vi "Data File Viewer.vi"(4 "error in (no error)":errorcluster, 6 "DataPlugin name":string, 7 "file path":path) -> (0 "error out":errorcluster, 2 "DataPlugin name out":string, 3 "file path out":path)   [LabVIEW 2020]
doc: "Opens the data file specified in the <B>file path</B> input and presents the data in the Data File Viewer dialog box."
uses:
  <vilib>/Utility/tdmsutil.llb/fileViewerConfigData.ctl
  <vilib>/Platform/storage/lvStorage.llb/_openFunction.ctl
  <vilib>/Platform/storage/Storage.llb/GetObjectFromID_Object.vi
panel:
  in  "Help":bool
  in  "Status":string
  in  "Quit":bool
  in  "Settings...":bool
  in  "Properties / Values / Graph":T1(tab)
  in  "Properties":i32(listbox)
  in  "Raw data values":i32(listbox)
  out "Waveform Graph":waveform(dbl)[](graph)
  in  "File contents":string(tree)
  # "Displaying values 1..1000"
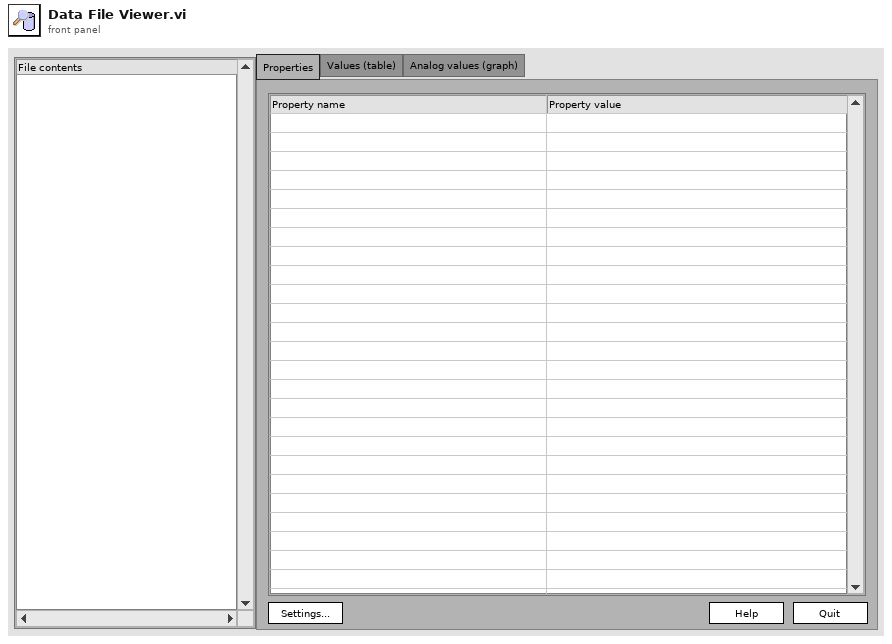
[diagram p1: front panel]
types:
  T1 = enum32{"Properties", "Values (table)", "Analog values (graph)"}
  T2 = typedef "_openFunction.ctl" = enum16{"open", "open or create", "create or replace", "create", "open (read only)"}
  T3 = typedef "fileViewerConfigData.ctl" = cluster{"Show all (table)":bool, "Show all (graph)":bool, "limit (table)":u64, "limit (graph)":u64, "no show":bool, "start (table)":u64, "start (graph)":u64}
  T4 = cluster{"Tree":refnum<vi>, "Tab Control":refnum<vi>, "property list":refnum<vi>, "raw data list":refnum<vi>, "Waveform Graph":refnum<vi>, "Ok":refnum<vi>, "Ok 2":refnum<vi>, "Ok 3":refnum<vi>, "Ok 4":refnum<vi>}
  T5 = typedef "usiPluginInformation.ctl" = cluster{"name":string, "version":string, "type":string, "read-only?":bool, "extensions":string[]}
  T6 = typedef "LVRectTypeDef.ctl" = cluster{"Left":i16, "Top":i16, "Right":i16, "Bottom":i16}
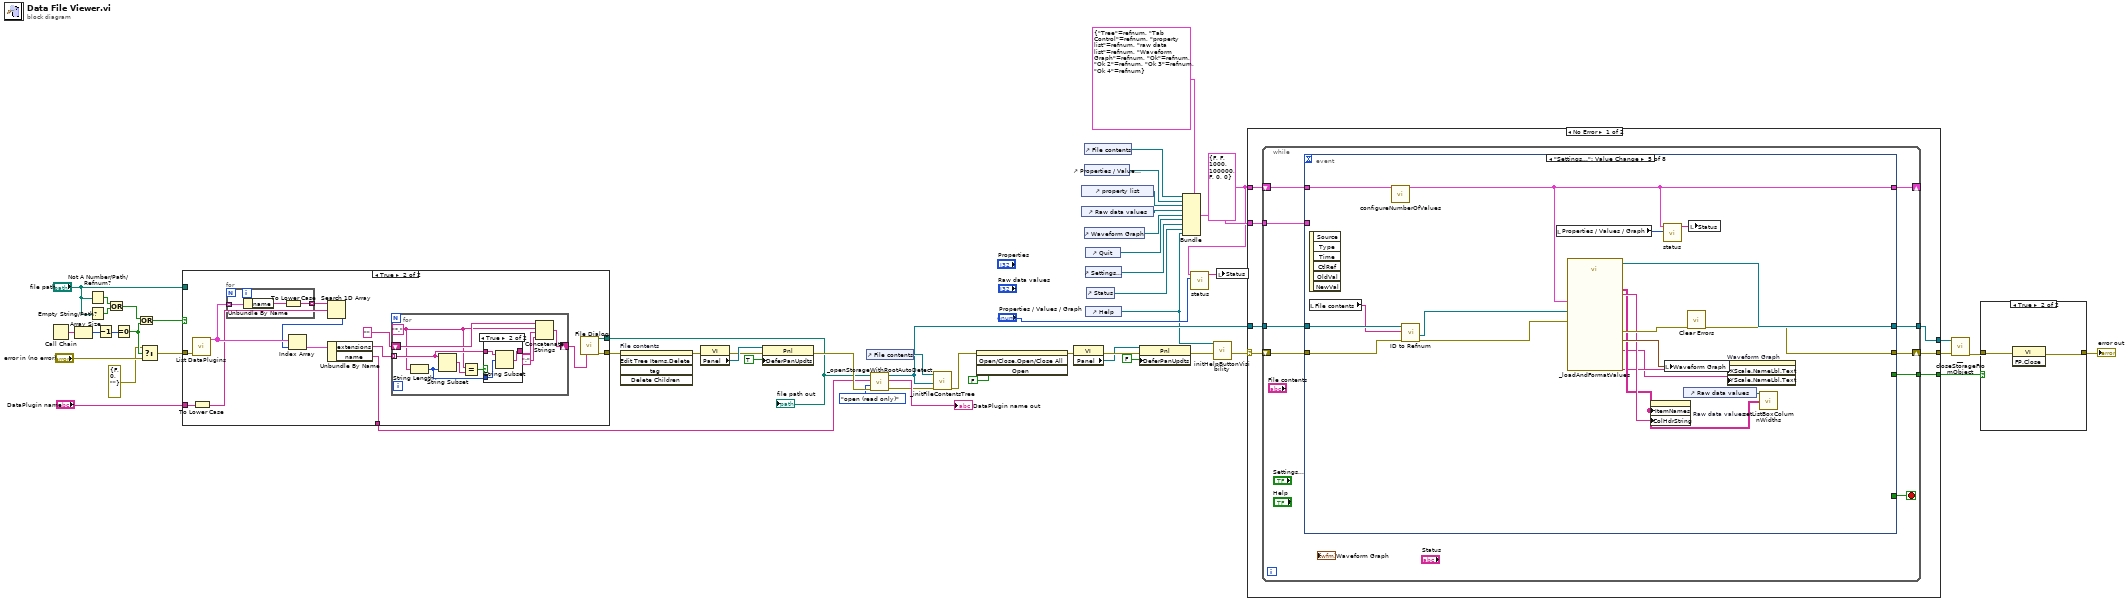
[diagram p0: block diagram]
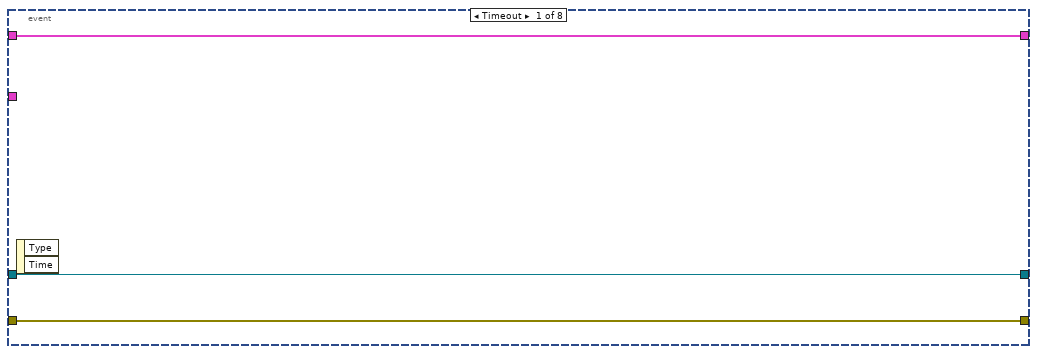
[diagram p5: hidden frame]
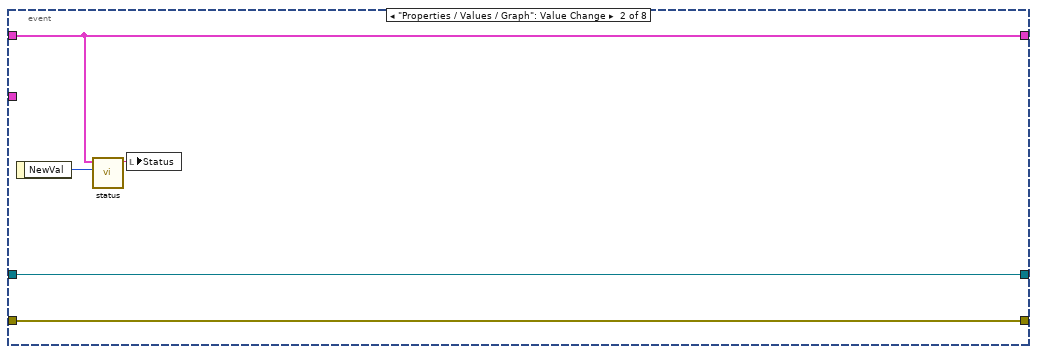
[diagram p6: hidden frame]
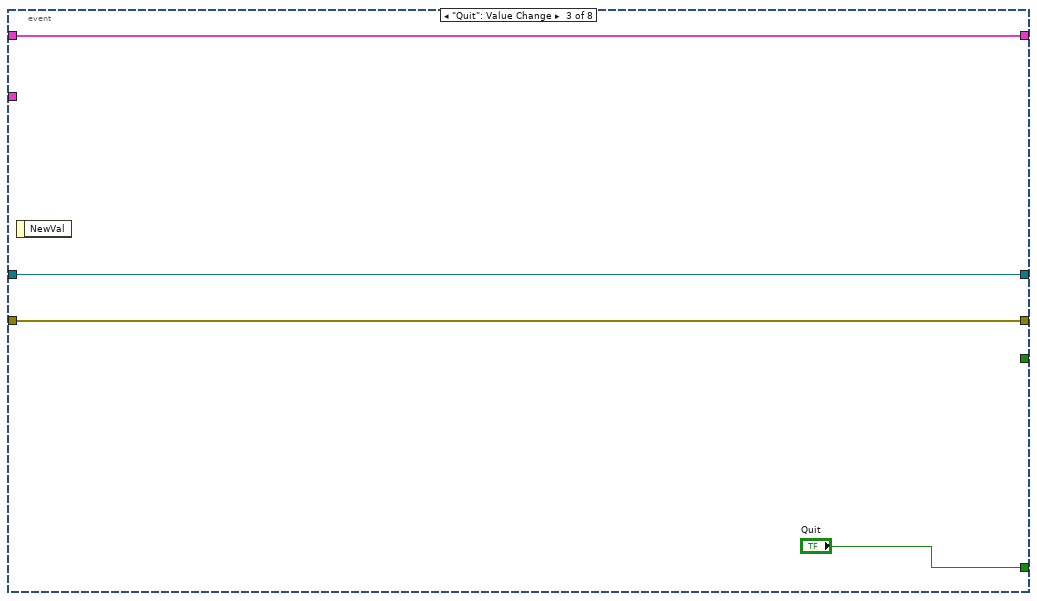
[diagram p7: hidden frame]
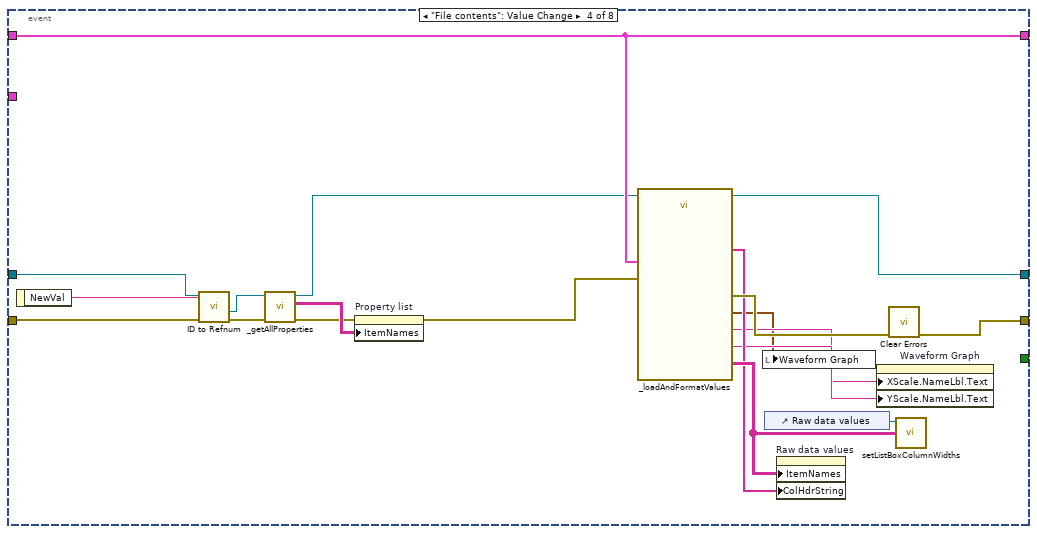
[diagram p8: hidden frame]
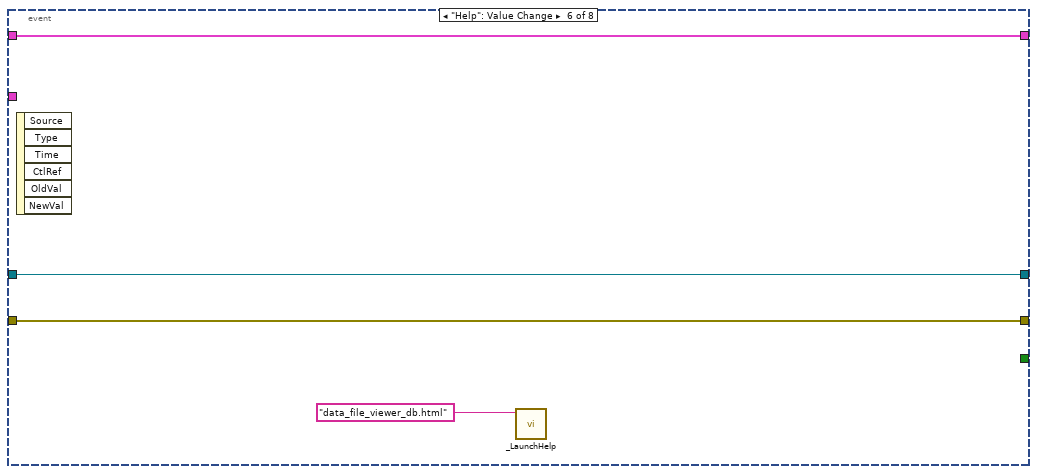
[diagram p9: hidden frame]
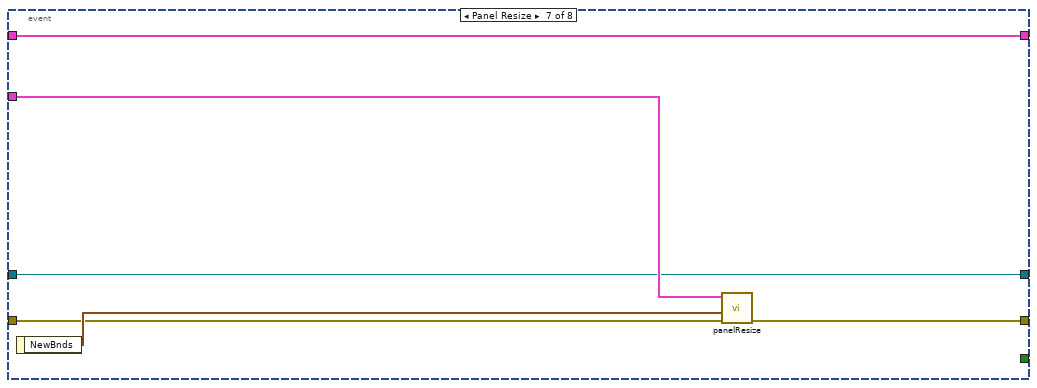
[diagram p10: hidden frame]
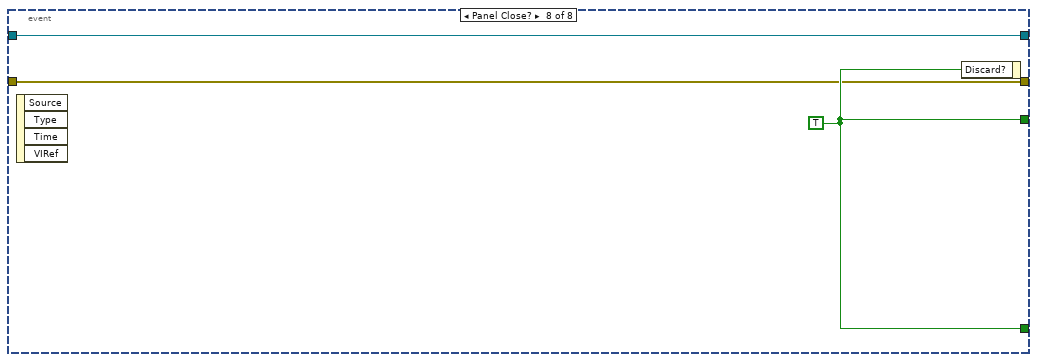
[diagram p11: hidden frame]
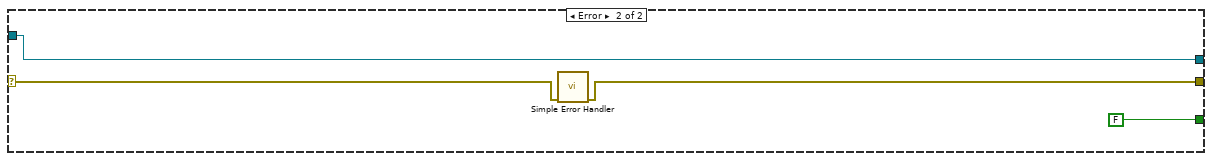
[diagram p12: hidden frame]
diagram:
  w31 = T3 {"Show all (table)"=FALSE, "Show all (graph)"=FALSE, "limit (table)"=1000, "limit (graph)"=100000, "no show"=FALSE, "start (table)"=0, "start (graph)"=0} ("TDMS File Viewer Configuration")
  n1 = Call Chain() -> (call chain=w24:string[])
  n2 = Array Size(array=w24) -> (size(s)=w22:i32)
  n3 = Not A Number/Path/Refnum?(number/path/refnum="file path") -> (NaN/Path/Refnum?=w26:bool)
  n4 = Empty String/Path?(string/path="file path") -> (empty?=w25:bool)
  n5 = Decrement(x=w22) -> (x-1=w21:i32)
  n6 = Or(x=w26, y=w25) -> (x .or. y?=w23:bool)
  n7 = Equal To 0?(x=w21) -> (x = 0?=w19:bool)
  n8 = Or(x=w23, y=w19) -> (x .or. y?=w20:bool)
  n9 = Select(t=errorcluster {"status"=FALSE, "code"=0, "source"=""}, s=w19, f="error in (no error)") -> (s? t:f=w18:errorcluster)
  n10 = case shown="True" w20 {
    tunnel: [w56 w69] -> w7
    tunnel: "file path" -> [w56 _]
    tunnel: [w55 w68] -> w15
    tunnel: w18 -> [w55 w67]
    tunnel: "DataPlugin name" -> [w54 w65]
    tunnel: [w54 w58] -> w8
    frame False {
    }
    frame True {
      n11 = call <vilib>:"List DataPlugins.vi"("error in (no error)"=w67) -> ("DataPlugin information"=w64:T5[])  [unwired: 13 in, 1 out]
      n12 = To Lower Case(string=w65) -> (all lower case string=w61:string)
      n13 = for {
        tunnel: w64 -> [w85] mode=indexing
        tunnel: [w84] -> w66 mode=indexing
        n14 = Unbundle By Name(w85) -> ("name"=w83:string)
        n15 = To Lower Case(string=w83) -> (all lower case string=w84:string)
      }
      n16 = Search 1D Array(1D array=w66, element=w61) -> (index of element=w63:i32)  [unwired: 1 in]
      n17 = Index Array(array=w64, index=w63) -> (element=w62:T5)
      n18 = Unbundle By Name(w62) -> ("extensions"=w60:string[], "name"=w58:string)
      n19 = for {
        tunnel: w60 -> [w73] mode=indexing
        shift-right: [w77] -> w57
        shift-left: "" -> [w76]
        w70 = "*." ("string")
        n20 = String Length(string=w70) -> (length=w71:i32)
        n21 = String Subset(string=w73, length (rest)=w71) -> (substring=w72:string)  [unwired: 1 in]
        n22 = Equal?(x=w70, y=w72) -> (x = y?=w74:bool)
        n23 = case shown="True" w74 {
          tunnel: [w79 w80] -> w78
          tunnel: w73 -> [w79 w82]
          tunnel: w71 -> [_ w81]
          frame False {
          }
          frame True {
            n24 = String Subset(string=w82, offset (0)=w81) -> (substring=w80:string)  [unwired: 1 in]
          }
        }
        n25 = Concatenate Strings(w76, w70, w78, ";" ("string")) -> (w77:string)
      }
      n26 = call "File Dialog"("pattern (all files)"=w57) -> ("selected path"=w69:path, "error out"=w68:errorcluster)  [unwired: 6 in, 7 out]
    }
  }
  "file path out" <- w7
  n27 = invoke on="File contents" class="Tree (strict)" method="Edit Tree Items.Delete"(error in=w15) -> (error out=w50:errorcluster)  [unwired: 4 in, 4 out]
  n28 = property class="VI"(error in=w50) -> (error out=w51:errorcluster, "Panel"=w52:refnum<vi>)  [unwired: 1 in, 1 out]
  n29 = property class="Pnl"(reference=w52, error in=w51, "DeferPanUpdts"=TRUE ("Defer Panel Updates")) -> (error out=w10:errorcluster)  [unwired: 1 out]
  n30 = control-ref of="File contents"() -> (w34:refnum<vi>)
  n31 = call <vilib>:"_openStorageWithRootAutoDetect.vi"("error in (no error)"=w10, "Overwrite Options"=_openFunction."open (read only)", "Storage Format"=w8, "Storage Location"=w7) -> ("error out"=w4:errorcluster, "Storage Format out"=→"DataPlugin name out":string, "Data Object"=w5:refnum<k20>)  [unwired: 5 in]
  n32 = call <vilib>:"_initFileContentsTree.vi"("error in (no error)"=w4, "File refnum in"=w5, "reference"=w34) -> ("error out"=w46:errorcluster)  [unwired: 4 in]
  n33 = invoke on="File contents" class="Tree (strict)" method="Open/Close.Open/Close All"(error in=w46, "Open"=FALSE ("Open?")) -> (error out=w45:errorcluster)  [unwired: 2 in, 3 out]
  n34 = property class="VI"(error in=w45) -> (error out=w48:errorcluster, "Panel"=w47:refnum<vi>)  [unwired: 1 in, 1 out]
  n35 = control-ref of="property list"() -> (w40:refnum<vi>)
  n36 = control-ref of="Raw data values"() -> (w39:refnum<vi>)
  n37 = control-ref of="Properties / Values / Graph"() -> (w41:refnum<vi>)
  n38 = control-ref of="Waveform Graph"() -> (w38:refnum<vi>)
  n39 = control-ref of="File contents"() -> (w43:refnum<vi>)
  n40 = control-ref of="Quit"() -> (w37:refnum<vi>)
  n41 = control-ref of="Settings..."() -> (w35:refnum<vi>)
  n42 = control-ref of="Help"() -> (w1:refnum<vi>)
  n43 = control-ref of="Status"() -> (w33:refnum<vi>)
  n44 = property class="Pnl"(reference=w47, error in=w48, "DeferPanUpdts"=FALSE ("Defer Panel Updates")) -> (error out=w2:errorcluster)  [unwired: 1 out]
  n45 = Bundle(cluster=T4 {"Tree"=refnum, "Tab Control"=refnum, "property list"=refnum, "raw data list"=refnum, "Waveform Graph"=refnum, "Ok"=refnum, "Ok 2"=refnum, "Ok 3"=refnum, "Ok 4"=refnum} ("control refs"), "Tree"=w43, "Tab Control"=w41, "property list"=w40, "raw data list"=w39, "Waveform Graph"=w38, "Ok"=w37, "Ok 2"=w35, "Ok 3"=w33, "Ok 4"=w1) -> (w42:T4)
  n46 = call <vilib>:"status.vi"("tab sheet"="Properties / Values / Graph", "TDMS File Viewer Configuration"=w31) -> ("status"=w32:string)  [unwired: 5 out]
  n47 = call <vilib>:"initHelpButtonVisibility.vi"("error in"=w2, "Help"=w1) -> ("error out"=w3:errorcluster)  [unwired: 9 in]
  n48 = local write "Status"(w32) -> ()
  n49 = case shown="No Error" w3 {
    selector: w3 -> [w89 w167]
    tunnel: [w92 w166] -> w13
    tunnel: w42 -> [w91 _]
    tunnel: w31 -> [w90 _]
    tunnel: [w88 FALSE] -> w29
    tunnel: w5 -> [w87 w164]
    tunnel: [w86 w164] -> w11
    frame No Error {
      n50 = while {
        shift-right: [w100] -> w92
        shift-left: w89 -> [w101]
        tunnel: w91 -> [w98]
        shift-right: [w96] -> _
        shift-left: w90 -> [w97]
        tunnel: [w95] -> w88
        tunnel: w87 -> [w94]
        tunnel: [w93] -> w86
        stop <- w99 stop-if-true
        n51 = event shown="[4] \"Settings...\": Value Change" {
          selector: _ -> [_ _ _ _ _ _ _ _]
          dyn-events: _ -> [_ _ _ _ _ _ _ _]
          timeout: _ -> [_ _ _ _ _ _ _ _]
          tunnel: w101 -> [w104 w109 w112 w116 w137 w153 w158 w161]
          tunnel: [w104 w109 w112 w129 w134 w153 w157 w161] -> w100
          tunnel: [_ _ "Quit" _ _ _ _ w163] -> w99
          tunnel: w98 -> [_ _ _ _ _ _ w159 _]
          tunnel: w97 -> [w103 w106 w111 w125 w150 w154 w156 _]
          tunnel: [w103 w106 w111 w125 w140 w154 w156 _] -> w96
          tunnel: [_ _ _ _ _ _ _ w163] -> w95
          tunnel: w94 -> [w102 w105 w110 w117 w138 w152 w155 w162]
          tunnel: [w102 w105 w110 w119 w139 w152 w155 w162] -> w93
          event Timeout {
            n52 = event-data() -> ()  [unwired: 3 out]
          }
          event "Properties / Values / Graph": Value Change {
            n53 = event-data() -> ("NewVal"=w108:T1)  [unwired: 1 out]
            n54 = call <vilib>:"status.vi"("tab sheet"=w108, "TDMS File Viewer Configuration"=w106) -> ("status"=w107:string)  [unwired: 5 out]
            n55 = local write "Status"(w107) -> ()
          }
          event "Quit": Value Change {
            n56 = event-data() -> ()  [unwired: 2 out]
          }
          event "File contents": Value Change {
            n57 = event-data() -> ("NewVal"=w118:string)  [unwired: 1 out]
            n58 = call-poly <vilib>:"ID to Refnum.vi"("error in (no error)"=w116, "Object id"=w118, "storage refnum"=w117) -> ("error out"=w115:errorcluster, "new storage refnum"=w114:refnum<k20>)  [unwired: 3 in]
            n59 = call <vilib>:"_getAllProperties.vi"("error in (no error)"=w115, "storage refnum"=w114) -> ("error out"=w122:errorcluster, "property name value"=w123:string[][], "storage refnum out"=w121:refnum<k20>)  [unwired: 7 in]
            n60 = property on="Property list" class="MCListbox (strict)"(error in=w122, "ItemNames"=w123) -> (error out=w120:errorcluster)  [unwired: 1 in, 1 out]
            n61 = call <vilib>:"_loadAndFormatValues.vi"("error in (no error)"=w120, "configuration"=w125, "storage refnum"=w121) -> ("error out"=w130:errorcluster, "graph y names"=w127:string, "graph x names"=w126:string, "storage refnum out"=w119:refnum<k20>, "waveform values"=w124:waveform(dbl)[], "table values"=w132:string[][], "table headers"=w128:string[])  [unwired: 2 in]
            n62 = local write "Waveform Graph"(w124) -> ()
            n63 = control-ref of="Raw data values"() -> (w131:refnum<vi>)
            n64 = property on="Raw data values" class="MCListbox (strict)"("ItemNames"=w132, "ColHdrString"=w128) -> ()  [unwired: 2 in, 2 out]
            n65 = property on="Waveform Graph" class="WFGraph (strict)"("XScale.NameLbl.Text"=w126, "YScale.NameLbl.Text"=w127) -> ()  [unwired: 2 in, 2 out]
            n66 = call <vilib>:"Clear Errors.vi"("error in (no error)"=w130) -> ("error out"=w129:errorcluster)  [unwired: 1 in, 5 out]
            n67 = call <vilib>:"setListBoxColumnWidths.vi"("table data"=w132, "MCListbox Refnum"=w131) -> ()  [unwired: 1 out]
          }
          event "Settings...": Value Change {
            n68 = event-data() -> ()  [unwired: 7 out]
            n69 = local read "File contents"() -> (w136:string)
            n70 = call <vilib>:"configureNumberOfValues.vi"("TDMS File Viewer Configuration"=w150) -> ("TDMS File Viewer Configuration Out"=w140:T3)  [unwired: 10 out]
            n71 = call-poly <vilib>:"ID to Refnum.vi"("error in (no error)"=w137, "Object id"=w136, "storage refnum"=w138) -> ("error out"=w135:errorcluster, "new storage refnum"=w133:refnum<k20>)  [unwired: 3 in]
            n72 = local read "Properties / Values / Graph"() -> (w141:T1)
            n73 = call <vilib>:"_loadAndFormatValues.vi"("error in (no error)"=w135, "configuration"=w140, "storage refnum"=w133) -> ("error out"=w149:errorcluster, "graph y names"=w144:string, "graph x names"=w143:string, "storage refnum out"=w139:refnum<k20>, "waveform values"=w148:waveform(dbl)[], "table values"=w145:string[][], "table headers"=w147:string[])  [unwired: 2 in]
            n74 = property on="Raw data values" class="MCListbox (strict)"("ItemNames"=w145, "ColHdrString"=w147) -> ()  [unwired: 2 in, 2 out]
            n75 = call <vilib>:"status.vi"("tab sheet"=w141, "TDMS File Viewer Configuration"=w140) -> ("status"=w142:string)  [unwired: 5 out]
            n76 = local write "Waveform Graph"(w148) -> ()
            n77 = control-ref of="Raw data values"() -> (w146:refnum<vi>)
            n78 = call <vilib>:"Clear Errors.vi"("error in (no error)"=w149) -> ("error out"=w134:errorcluster)  [unwired: 5 in, 1 out]
            n79 = local write "Status"(w142) -> ()
            n80 = property on="Waveform Graph" class="WFGraph (strict)"("XScale.NameLbl.Text"=w143, "YScale.NameLbl.Text"=w144) -> ()  [unwired: 2 in, 2 out]
            n81 = call <vilib>:"setListBoxColumnWidths.vi"("table data"=w145, "MCListbox Refnum"=w146) -> ()  [unwired: 1 out]
          }
          event "Help": Value Change {
            n82 = event-data() -> ()  [unwired: 7 out]
            n83 = call <helpdir>:"_LaunchHelp.vi"("HTML filename"="data_file_viewer_db.html") -> ()  [unwired: 2 in, 5 out]
          }
          event Panel Resize {
            n84 = event-data() -> ("NewBnds"=w160:T6)  [unwired: 1 out]
            n85 = call <vilib>:"panelResize.vi"("error in (no error)"=w158, "NewBnds"=w160, "control refs"=w159) -> ("error out"=w157:errorcluster)  [unwired: 4 out]
          }
          event Panel Close? {
            w163 = TRUE
            n86 = event-data() -> ()  [unwired: 5 out]
            n87 = event-data("Discard?"=w163) -> ()  [unwired: 1 in, 1 out]
          }
        }
      }
    }
    frame Error {
      n88 = call <vilib>:"Simple Error Handler.vi"("error in (no error)"=w167) -> ("error out"=w166:errorcluster)  [unwired: 1 in, 7 out]
    }
  }
  n89 = call <vilib>:"__closeStorageFromObject.vi"("error in (no error)"=w13, "storage refnum"=w11) -> ("error out"=w12:errorcluster)  [unwired: 5 in]
  n90 = case shown="True" w29 {
    tunnel: w12 -> [w168 w170]
    tunnel: [w168 w169] -> w28
    frame False {
    }
    frame True {
      n91 = invoke class="VI" method="FP.Close"(error in=w170) -> (error out=w169:errorcluster)  [unwired: 2 in, 2 out]
    }
  }
  "error out" <- w28
